vi "Instance.vi"(10 "error in (no error)":errorcluster) -> (2 "error out":errorcluster, 3 "Device Manager":refnum<class "DeviceManager.lvclass">)   [LabVIEW 2020, in "PicoG-Core.lvlib" / "DeviceManager.lvclass"]
uses:
  DeviceManager.lvclass
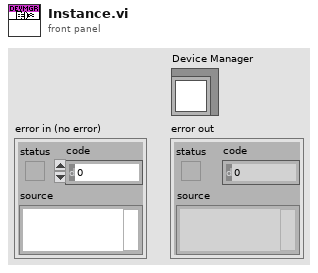
[diagram p1: front panel]
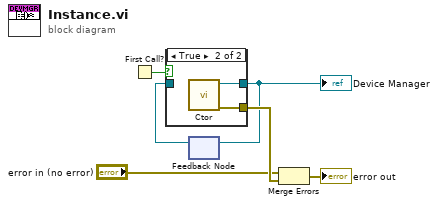
[diagram p0: block diagram]
diagram:
  n1 = First Call?() -> (First Call?: T/F=w2:bool)
  n2 = feedback #1() -> (w3:refnum<class "DeviceManager.lvclass">)  [unwired: 1 in]
  n3 = case shown="True" w2 {
    tunnel: [w7 w9] -> w4
    tunnel: w3 -> [w7 _]
    tunnel: [_ w8] -> w6
    frame False {
    }
    frame True {
      n4 = call "Ctor.vi"() -> ("error out"=w8:errorcluster, "DeviceManager out"=w9:refnum<class "DeviceManager.lvclass">)  [unwired: 10 in]
    }
  }
  "Device Manager" <- w4
  n5 = feedback-in #1(w4) -> ()
  n6 = Merge Errors("error in (no error)", w6) -> (→"error out":errorcluster)
